vi "convert timespec 64 to timespec 32.vi"(11 "timespec 64":cluster{"sec":u64, "nsec":u64}) -> (3 "timespec 32":cluster{"sec":u32, "nsec":u32})   [LabVIEW 2013, in "Linux RT Utilities.lvlib"]
uses:
  Linux RT Utilities.lvlib
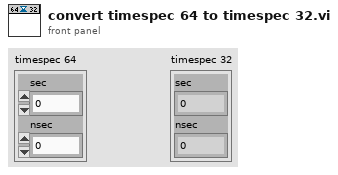
[diagram p1: front panel]
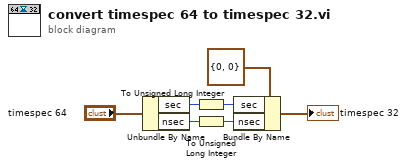
[diagram p0: block diagram]
diagram:
  n1 = Unbundle By Name("timespec 64") -> ("sec"=w4:u64, "nsec"=w3:u64)
  n2 = To Unsigned Long Integer(number=w4) -> (unsigned 32bit integer=w1:u32)
  n3 = To Unsigned Long Integer(number=w3) -> (unsigned 32bit integer=w2:u32)
  n4 = Bundle By Name(cluster=cluster{"sec":u32, "nsec":u32} {"sec"=0, "nsec"=0} ("timespec"), "sec"=w1, "nsec"=w2) -> (→"timespec 32":cluster{"sec":u32, "nsec":u32})
